vi "NXT_HINDBRAIN Translate Motor Command.vi"(1 "_motorCommands":T3, 2 "Tugboat Properties":T1={"_name"="Enterprise", "_pitch"=440, "_rudderCenter"=1450, "_propCenter"=1500, "_irServoCenter"=1600, "_rudderMin"=800, "_rudderMax"=2000, "_propMin"=1000, "_propMax"=2000, "_irServoMin"=800, "_irServoMax"=2200}) -> (0 "_motorData":T2)   [LabVIEW 2012, in "Tugboat.lvrbt"]
uses:
  Tugboat.lvrbt
  motorCommands_t.ctl
  motorData_t.ctl
  tugProperties_t.ctl
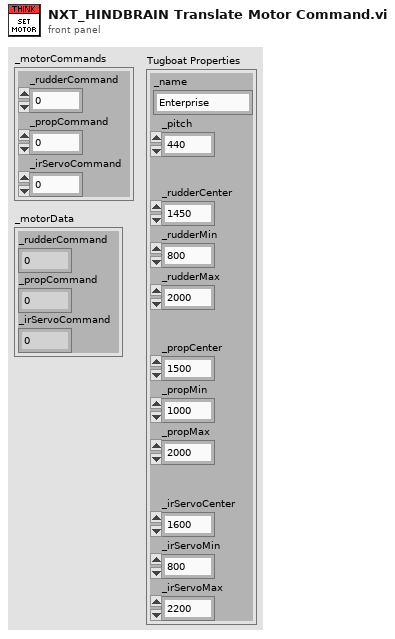
[diagram p1: front panel]
types:
  T1 = typedef "tugProperties_t.ctl" = cluster{"_name":string, "_pitch":i32, "_rudderCenter":u16, "_propCenter":u16, "_irServoCenter":u16, "_rudderMin":u16, "_rudderMax":u16, "_propMin":u16, "_propMax":u16, "_irServoMin":u16, "_irServoMax":u16}
  T2 = typedef "motorData_t.ctl" = cluster{"_rudderCommand":u16, "_propCommand":u16, "_irServoCommand":u16}
  T3 = typedef "motorCommands_t.ctl" = cluster{"_rudderCommand":i8, "_propCommand":i8, "_irServoCommand":i8}
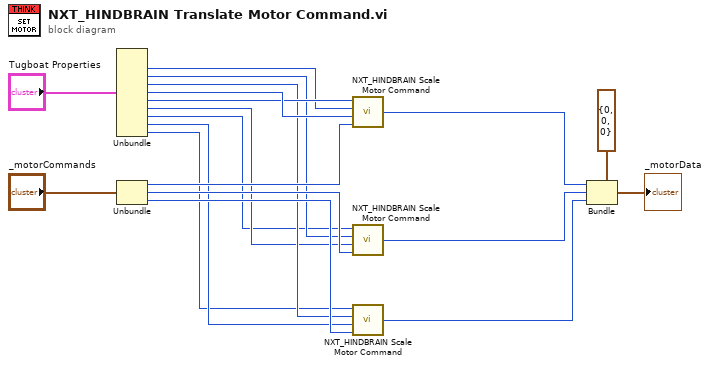
[diagram p0: block diagram]
diagram:
  n1 = Unbundle("Tugboat Properties") -> ("_rudderCenter"=w13:u16, "_propCenter"=w8:u16, "_irServoCenter"=w7:u16, "_rudderMin"=w15:u16, "_rudderMax"=w14:u16, "_propMin"=w6:u16, "_propMax"=w5:u16, "_irServoMin"=w4:u16, "_irServoMax"=w3:u16)  [unwired: 2 out]
  n2 = Unbundle("_motorCommands") -> ("_rudderCommand"=w11:i8, "_propCommand"=w10:i8, "_irServoCommand"=w9:i8)
  n3 = call "NXT_HINDBRAIN Scale Motor Command.vi"("command"=w11, "min"=w15, "mid"=w13, "max"=w14) -> ("converted"=w12:u16)
  n4 = call "NXT_HINDBRAIN Scale Motor Command.vi"("command"=w10, "min"=w6, "mid"=w8, "max"=w5) -> ("converted"=w2:u16)
  n5 = call "NXT_HINDBRAIN Scale Motor Command.vi"("command"=w9, "min"=w4, "mid"=w7, "max"=w3) -> ("converted"=w1:u16)
  n6 = Bundle(cluster=T2 {"_rudderCommand"=0, "_propCommand"=0, "_irServoCommand"=0} ("_motorData 2"), "_rudderCommand"=w12, "_propCommand"=w2, "_irServoCommand"=w1) -> (→"_motorData":T2)
